vi "Register gRPC Methods.vi"(8 "error in (no error)":errorcluster, 11 "Template Server in":refnum<class "ctet_mux.lvclass">) -> (0 "error out":errorcluster, 3 "Template Server out":refnum<class "ctet_mux.lvclass">)   [LabVIEW 2019, in "ctet_mux.lvlib" / "ctet_mux.lvclass"]
uses:
  ctet_mux.lvclass
  typeDefs/Server Internal UEs.ctl
  typeDefs/Server Internal Message.ctl
  typeDefs/Server gRPC UEs.ctl
  gRPC lvSupport/Server API/typeDefs/gRPCId Cluster.ctl
  gRPC lvSupport/Server API/typeDefs/grpcId.ctl
  ctet_mux.lvclass/ctet_mux.ctl
  gRPC lvSupport/gprc-lvsupport.lvlib
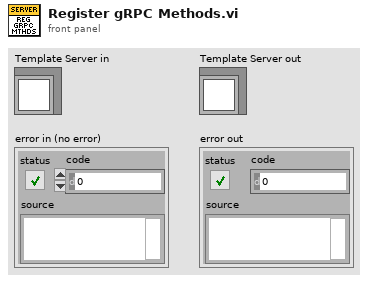
[diagram p1: front panel]
types:
  T1 = typedef "ctet_mux.lvlib/ctet_mux.lvclass/Server gRPC UEs.ctl" = cluster{"Invoke gRPC UE":refnum<user-event>, "Query gRPC UE":refnum<user-event>, "Register gRPC UE":refnum<user-event>, "OpenMUXSession gRPC UE":refnum<user-event>, "CloseMUXChannel gRPC UE":refnum<user-event>, "OpenMUXChannel gRPC UE":refnum<user-event>, "DisconnectAllMUXChannels gRPC UE":refnum<user-event>, "CloseMUXSession gRPC UE":refnum<user-event>, "ResetMUX gRPC UE":refnum<user-event>}
  T2 = typedef "ctet_mux.lvlib/ctet_mux.lvclass/Server Internal UEs.ctl" = cluster{"Invoke Internal UE":refnum<user-event>, "Query Internal UE":refnum<user-event>, "Register Internal UE":refnum<user-event>, "OpenMUXSession Internal UE":refnum<user-event>, "CloseMUXChannel Internal UE":refnum<user-event>, "OpenMUXChannel Internal UE":refnum<user-event>, "DisconnectAllMUXChannels Internal UE":refnum<user-event>, "CloseMUXSession Internal UE":refnum<user-event>, "ResetMUX Internal UE":refnum<user-event>}
  T3 = typedef "ctet_mux.lvlib/gprc-lvsupport.lvlib/grpcId.ctl" = u64
  T4 = typedef "ctet_mux.lvlib/ctet_mux.lvclass/Server Internal Message UE.ctl" = refnum<user-event>
  T5 = typedef "ctet_mux.lvlib/gprc-lvsupport.lvlib/gRPCId Cluster UE.ctl" = refnum<user-event>
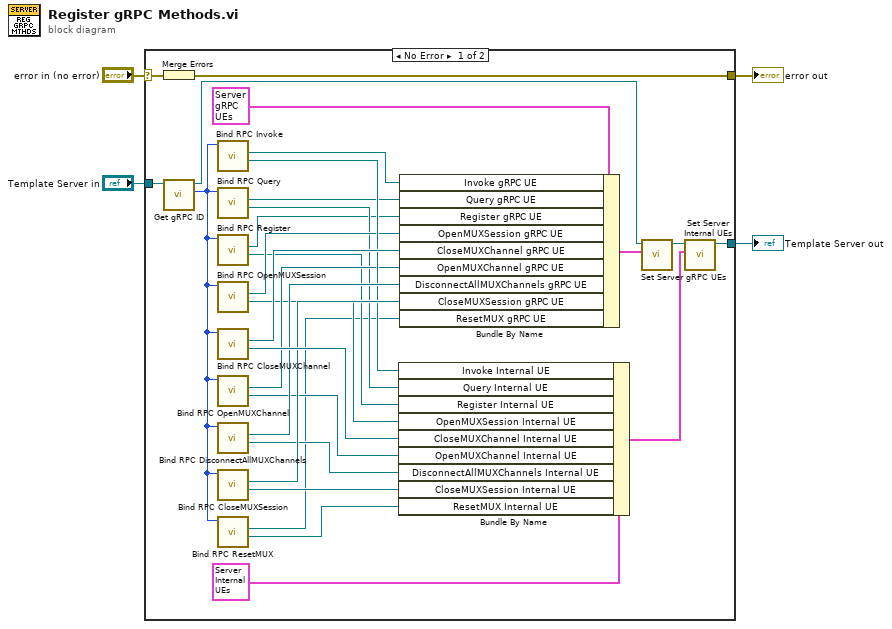
[diagram p0: block diagram]
diagram:
  n1 = case shown="No Error" "error in (no error)" {
    selector: "error in (no error)" -> [w24 w34]
    tunnel: "Template Server in" -> [w32 w35]
    tunnel: [w31 w34] -> w3
    tunnel: [w30 w35] -> w2
    frame No Error {
      n2 = Merge Errors(w24) -> (w31:errorcluster)
      n3 = call "Get gRPC ID.vi"("OOP Server in"=w32) -> ("gRPC ID"=w23:T3, "OOP Server out"=w33:refnum<class "ctet_mux.lvclass">)  [unwired: 9 in]
      n4 = call "Bind RPC Invoke.vi"("gRPCid server in"=w23) -> ("Invoke Internal UE"=w16:T4, "Invoke gRPC UE"=w15:T5)  [unwired: 7 in, 2 out]
      n5 = call "Bind RPC Query.vi"("gRPCid server in"=w23) -> ("Query Internal UE"=w10:T4, "Query gRPC UE"=w9:T5)  [unwired: 7 in, 2 out]
      n6 = call "Bind RPC Register.vi"("gRPCid server in"=w23) -> ("Register Internal UE"=w8:T4, "Register gRPC UE"=w7:T5)  [unwired: 7 in, 2 out]
      n7 = call "Bind RPC OpenMUXSession.vi"("gRPCid server in"=w23) -> ("OpenMUXSession Internal UE"=w12:T4, "OpenMUXSession gRPC UE"=w11:T5)  [unwired: 7 in, 2 out]
      n8 = call "Bind RPC CloseMUXChannel.vi"("gRPCid server in"=w23) -> ("CloseMUXChannel Internal UE"=w22:T4, "CloseMUXChannel gRPC UE"=w21:T5)  [unwired: 7 in, 2 out]
      n9 = call "Bind RPC OpenMUXChannel.vi"("gRPCid server in"=w23) -> ("OpenMUXChannel Internal UE"=w14:T4, "OpenMUXChannel gRPC UE"=w13:T5)  [unwired: 7 in, 2 out]
      n10 = call "Bind RPC DisconnectAllMUXChannels.vi"("gRPCid server in"=w23) -> ("DisconnectAllMUXChannels Internal UE"=w18:T4, "DisconnectAllMUXChannels gRPC UE"=w17:T5)  [unwired: 7 in, 2 out]
      n11 = call "Bind RPC CloseMUXSession.vi"("gRPCid server in"=w23) -> ("CloseMUXSession Internal UE"=w20:T4, "CloseMUXSession gRPC UE"=w19:T5)  [unwired: 7 in, 2 out]
      n12 = call "Bind RPC ResetMUX.vi"("gRPCid server in"=w23) -> ("ResetMUX Internal UE"=w6:T4, "ResetMUX gRPC UE"=w5:T5)  [unwired: 7 in, 2 out]
      n13 = Bundle By Name ("Bundle Internal UEs")(cluster=T2 {"Invoke Internal UE"=refnum, "Query Internal UE"=refnum, "Register Internal UE"=refnum, "OpenMUXSession Internal UE"=refnum, "CloseMUXChannel Internal UE"=refnum, "OpenMUXChannel Internal UE"=refnum, "DisconnectAllMUXChannels Internal UE"=refnum, "CloseMUXSession Internal UE"=refnum, "ResetMUX Internal UE"=refnum} ("Server Internal UEs"), "Invoke Internal UE"=w16, "Query Internal UE"=w10, "Register Internal UE"=w8, "OpenMUXSession Internal UE"=w12, "CloseMUXChannel Internal UE"=w22, "OpenMUXChannel Internal UE"=w14, "DisconnectAllMUXChannels Internal UE"=w18, "CloseMUXSession Internal UE"=w20, "ResetMUX Internal UE"=w6) -> (w29:T2)
      n14 = Bundle By Name ("Bundle gRPC UEs")(cluster=T1 {"Invoke gRPC UE"=refnum, "Query gRPC UE"=refnum, "Register gRPC UE"=refnum, "OpenMUXSession gRPC UE"=refnum, "CloseMUXChannel gRPC UE"=refnum, "OpenMUXChannel gRPC UE"=refnum, "DisconnectAllMUXChannels gRPC UE"=refnum, "CloseMUXSession gRPC UE"=refnum, "ResetMUX gRPC UE"=refnum} ("gRPC Server Method Events"), "Invoke gRPC UE"=w15, "Query gRPC UE"=w9, "Register gRPC UE"=w7, "OpenMUXSession gRPC UE"=w11, "CloseMUXChannel gRPC UE"=w21, "OpenMUXChannel gRPC UE"=w13, "DisconnectAllMUXChannels gRPC UE"=w17, "CloseMUXSession gRPC UE"=w19, "ResetMUX gRPC UE"=w5) -> (w26:T1)
      n15 = call "Set Server gRPC UEs.vi"("Server gRPC UEs"=w26, "OOP Server in"=w33) -> ("OOP Server out"=w27:refnum<class "ctet_mux.lvclass">)  [unwired: 9 in]
      n16 = call "Set Server Internal UEs.vi"("Server Internal UEs"=w29, "OOP Server in"=w27) -> ("OOP Server out"=w30:refnum<class "ctet_mux.lvclass">)  [unwired: 9 in]
    }
    frame Error {
    }
  }
  "error out" <- w3
  "Template Server out" <- w2
